vi "CLSUIP_GetUnwiredTerminals.vi"(8 "error in (no error)":errorcluster, 11 "Growable Node Ref":refnum<vi>) -> (0 "error out":errorcluster, 2 "Unwired Terminals":refnum<vi>[](array[refnum]), 3 "Growable Node Ref out":refnum<vi>)   [LabVIEW 2021, in "MemberVICreation.lvlib"]
uses:
  <resource>/Framework/Providers/LVClassLibrary/NewAccessors/MemberVICreation.lvlib
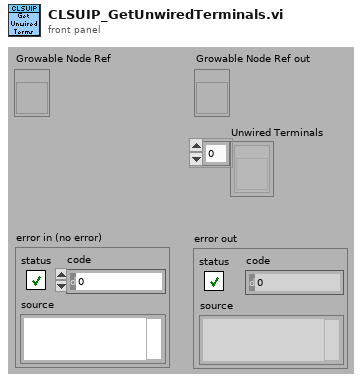
[diagram p1: front panel]
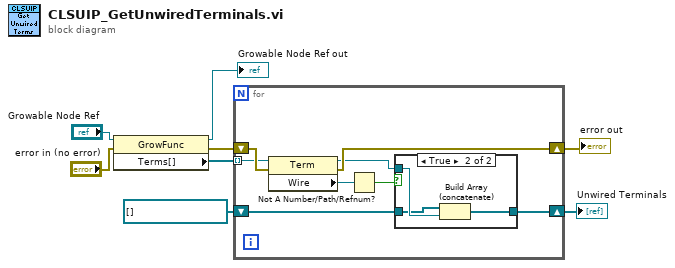
[diagram p0: block diagram]
diagram:
  n1 = property class="GrowFunc"(reference="Growable Node Ref", error in="error in (no error)") -> (reference out=→"Growable Node Ref out":refnum<vi>, error out=w5:errorcluster, "Terms[]"=w6:refnum<vi>[])
  n2 = for {
    tunnel: w6 -> [w15] mode=indexing
    shift-right: [w12] -> w4
    shift-left: w5 -> [w16]
    shift-right: [w9] -> w1
    shift-left: refnum<vi>[] [] -> [w10]
    n3 = property class="Term"(reference=w15, error in=w16) -> (reference out=w11:refnum<vi>, error out=w12:errorcluster, "Wire"=w14:refnum<vi>)
    n4 = Not A Number/Path/Refnum?(number/path/refnum=w14) -> (NaN/Path/Refnum?=w13:bool)
    n5 = case shown="True" w13 {
      tunnel: w11 -> [_ w20]
      tunnel: w10 -> [w17 w19]
      tunnel: [w17 w18] -> w9
      frame False {
      }
      frame True {
        n6 = Build Array (concatenate)(w19, w20) -> (w18:refnum<vi>[])
      }
    }
  }
  "error out" <- w4
  "Unwired Terminals" <- w1
